vi "M03 Hybrid Car.vi"   [LabVIEW 2016]
types:
  T1 = typedef "LVHSConnector.ctl" = refnum<class "BrickReference.lvclass">
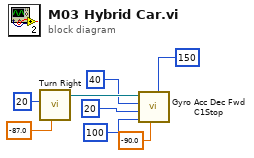
[diagram p0: block diagram]
diagram:
  n1 = call "Turn Right.vi"("Turning angle"=sgl -87.0, "Motor B (right)"=i8 20) -> ("EV3 out"=w6:T1)  [unwired: 9 in]
  n2 = call "Gyro Acc Dec Fwd C1Stop.vi"("Threshold to C1"=150, "Ini. Degrees"=sgl -90.0, "Threshold to De-acc"=100, "De-acc"=20, "Acc"=40, "EV3 in"=w6) -> ()  [unwired: 5 in, 1 out]
